vi "Diff_Drive_System_Set_Speed_Target.vi"(9 "Right Speed Target FT/S":dbl, 11 "Left Speed Target FT/S":dbl) -> ()   [LabVIEW 2019]
uses:
  Diff_Drive_System_Globals.vi
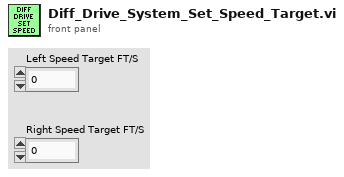
[diagram p1: front panel]
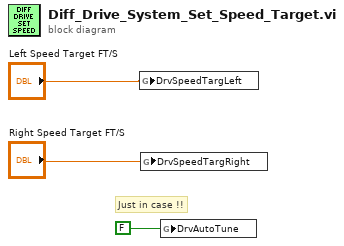
[diagram p0: block diagram]
diagram:
  # "Just in case !!"
  n1 = global write "Diff_Drive_System_Globals.vi" "DrvSpeedTargLeft"("Left Speed Target FT/S") -> ()
  n2 = global write "Diff_Drive_System_Globals.vi" "DrvSpeedTargRight"("Right Speed Target FT/S") -> ()
  n3 = global write "Diff_Drive_System_Globals.vi" "DrvAutoTune"(FALSE ("AutoTune")) -> ()
